vi "Newton Raphson Inner Part.vi"(1 "table":i32[][](array[numeric]), 4 "accuracy":dbl format="%.2f", 5 "end/start":dbl format="%.2f", 6 "case":bool, 7 "start/end":dbl format="%.2f", 8 "h":dbl format="%.2f", 9 "result":dbl[](array[numeric]) format="%.2f", 10 "list of variables":i32[](array[numeric])) -> (0 "error":i32, 2 "zero":dbl format="%.2f", 3 "f(zero)":dbl format="%.2f")   [LabVIEW 2018, in "NI_Gmath.lvlib"]
uses:
  NI_Gmath.lvlib
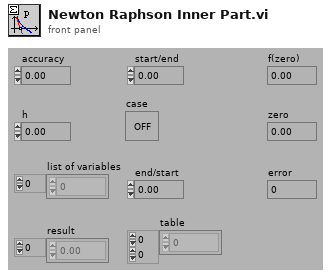
[diagram p1: front panel]
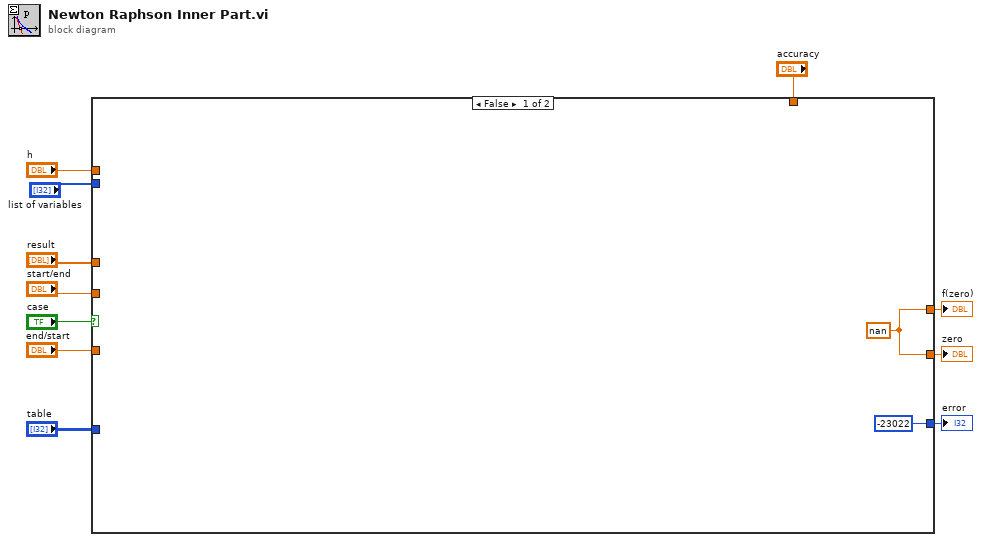
[diagram p0: block diagram]
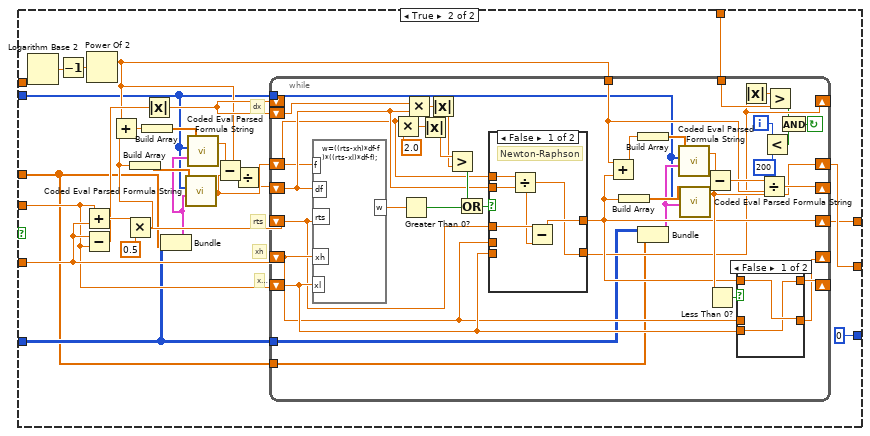
[diagram p2: hidden frame]
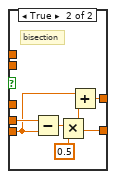
[diagram p4: hidden frame]
diagram:
  n1 = case shown="False" "case" {
    tunnel: [w13 w39] -> w2
    tunnel: [w13 w38] -> w1
    tunnel: "end/start" -> [_ w37]
    tunnel: "start/end" -> [_ w36]
    tunnel: "h" -> [_ w22]
    tunnel: "accuracy" -> [_ w21]
    tunnel: [-23022 0] -> w6
    tunnel: "list of variables" -> [_ w16]
    tunnel: "table" -> [_ w15]
    tunnel: "result" -> [_ w14]
    frame False {
      w13 = nan
    }
    frame True {
      # "rts"
      # "dx"
      # "xh"
      # "xl"
      n2 = Logarithm Base 2(1:w22) -> (0:w25:dbl)
      n3 = Decrement(x=w25) -> (x-1=w24:dbl)
      n4 = Add(x=w36, y=w37) -> (x+y=w34:dbl)
      n5 = Subtract(x=w37, y=w36) -> (x-y=w33:dbl)
      n6 = Power Of 2(x=w24) -> (2^x=w23:dbl)
      n7 = Multiply(x=w34, y=0.5) -> (x*y=w31:dbl)
      n8 = Add(x=w23, y=w31) -> (x+y=w30:dbl)
      n9 = Build Array(w31) -> (w19:dbl[])
      n10 = Build Array(w30) -> (w18:dbl[])
      n11 = Absolute Value(x=w33) -> (abs(x)=w32:dbl)
      n12 = Bundle("table"=w15, "result"=w14) -> (w17:cluster{"table":i32[][], "result":dbl[]})  [unwired: 1 in]
      n13 = call "Coded Eval Parsed Formula String.vi"("Parsed Formula"=w17, "Variables"=w16, "X Values"=w19) -> ("y value"=w28:dbl)  [unwired: 1 in, 1 out]
      n14 = call "Coded Eval Parsed Formula String.vi"("Parsed Formula"=w17, "Variables"=w16, "X Values"=w18) -> ("y value"=w29:dbl)  [unwired: 1 in, 1 out]
      n15 = Subtract(x=w29, y=w28) -> (x-y=w27:dbl)
      n16 = Divide(x=w27, y=w23) -> (x/y=w26:dbl)
      n17 = while {
        tunnel: w14 -> [w40]
        tunnel: w15 -> [w41]
        tunnel: w16 -> [w42]
        tunnel: w23 -> [w57]
        tunnel: w21 -> [w63]
        shift-left: w32 -> [w62]
        shift-left: w36 -> [w69]
        shift-right: [w67] -> _
        shift-left: w37 -> [w68]
        shift-right: [w66] -> _
        shift-left: w26 -> [w71]
        shift-right: [w56] -> _
        shift-left: w28 -> [w65]
        shift-right: [w55] -> w39
        shift-left: w32 -> [_]
        shift-right: [w52] -> _
        shift-left: w31 -> [w64]
        shift-right: [w54] -> w38
        i -> [w50]
        stop <- w46 continue-if-true
        n18 = formula code="w=((rts-xh)*df-f)*((rts-xl)*df-f);"("f"=w65, "df"=w71, "rts"=w64, "xh"=w68, "xl"=w69) -> ("w"=w51:dbl)
        n19 = Multiply(x=w65, y=2.0) -> (x*y=w76:dbl)
        n20 = Greater Than 0?(x=w51) -> (x > 0?=w53:bool)
        n21 = Multiply(x=w62, y=w71) -> (x*y=w77:dbl)
        n22 = Absolute Value(x=w76) -> (abs(x)=w75:dbl)
        n23 = Absolute Value(x=w77) -> (abs(x)=w74:dbl)
        n24 = Greater?(x=w75, y=w74) -> (0:w73:bool)
        n25 = Or(x=w73, y=w53) -> (x .or. y?=w72:bool)
        n26 = case shown="False" w72 {
          tunnel: w68 -> [_ w93]
          tunnel: w69 -> [_ w89]
          tunnel: [w83 w90] -> w52
          tunnel: [w84 w88] -> w54
          tunnel: w65 -> [w87 _]
          tunnel: w71 -> [w86 _]
          tunnel: w64 -> [w85 _]
          frame False {
            # "Newton-Raphson"
            n27 = Divide(x=w87, y=w86) -> (x/y=w83:dbl)
            n28 = Subtract(x=w85, y=w83) -> (x-y=w84:dbl)
          }
          frame True {
            # "bisection"
            n29 = Subtract(x=w93, y=w89) -> (x-y=w92:dbl)
            n30 = Multiply(x=w92, y=0.5) -> (x*y=w90:dbl)
            n31 = Add(x=w89, y=w90) -> (x+y=w88:dbl)
          }
        }
        n32 = Add(x=w57, y=w54) -> (x+y=w60:dbl)
        n33 = Build Array(w54) -> (w44:dbl[])
        n34 = Build Array(w60) -> (w45:dbl[])
        n35 = Bundle("table"=w41, "result"=w40) -> (w43:cluster{"table":i32[][], "result":dbl[]})  [unwired: 1 in]
        n36 = call "Coded Eval Parsed Formula String.vi"("Parsed Formula"=w43, "Variables"=w42, "X Values"=w45) -> ("y value"=w59:dbl)  [unwired: 1 in, 1 out]
        n37 = call "Coded Eval Parsed Formula String.vi"("Parsed Formula"=w43, "Variables"=w42, "X Values"=w44) -> ("y value"=w55:dbl)  [unwired: 1 in, 1 out]
        n38 = Subtract(x=w59, y=w55) -> (x-y=w58:dbl)
        n39 = Less Than 0?(x=w55) -> (x < 0?=w70:bool)
        n40 = case shown="False" w70 {
          tunnel: w69 -> [w79 _]
          tunnel: w68 -> [_ w81]
          tunnel: w54 -> [w80 w82]
          tunnel: [w79 w82] -> w67
          tunnel: [w80 w81] -> w66
          frame False {
          }
          frame True {
          }
        }
        n41 = Absolute Value(x=w52) -> (abs(x)=w61:dbl)
        n42 = Divide(x=w58, y=w57) -> (x/y=w56:dbl)
        n43 = Less?(x=w50, y=200) -> (x < y?=w48:bool)
        n44 = Greater?(x=w61, y=w63) -> (0:w47:bool)
        n45 = And(x=w47, y=w48) -> (x .and. y?=w46:bool)
      }
    }
  }
  "error" <- w6
  "zero" <- w2
  "f(zero)" <- w1
